vi "Servo.vi"() -> ()   [LabVIEW 2017]
uses:
  <vilib>/Platform/TimedLoop/XDataNode/timing_clust.ctl
  <vilib>/Platform/TimedLoop/XDataNode/nitl_modes.ctl
  <vilib>/Platform/TimedLoop/XDataNode/wakeup.ctl
  <vilib>/rvi/FXPMathLib/basic elements/FxpIntAccumulator/subVIs/nifxpmath_IntAccumulator_SimConfig.ctl
  <vilib>/rvi/Emulation/niFpgaGetClockAttributes.vi
  <vilib>/rvi/Emulation/niFpgaSctlEmulationGetInTimedLoop.vi
  <vilib>/rvi/Emulation/niFpgaEmulationReportErrorSimple.vi
  <vilib>/rvi/eio/common/nirviEmuTemplateMethod_errors.vi
  <vilib>/rvi/Emulation/niFpgaCriticalErrorInLSC.vi
  <vilib>/rvi/Analysis/common/codeGenErrors/XNode/niFpgaXNodeCodeGenErrorHandle.vi
  <vilib>/rvi/FXPMathLib/basic elements/FxpIntAccumulator/simVIs/DllFxpIntAccumulator_sub.vi
  <vilib>/eio/EIONode/EIONode.xnode
  <vilib>/rvi/Analysis/measure/dc-rms/XNode/niFpgaDC-RMS.xnode
  <vilib>/Platform/TimedLoop/XDataNode/XDataNode.xnode
  <vilib>/rvi/FXPMathLib/basic elements/FxpIntAccumulator/XNode/nifxpmath_IntAccumulator.xnode
  <vilib>/rvi/FXPMathLib/FxpMul/XNode/nifxpmath_Multiplier.xnode
  <vilib>/Platform/TimedLoop/XDataNode/XDNodeRunTimeDep.lvlib
  <vilib>/rvi/FXPMathLib/sim/FxpSim.dll
panel:
  out "Forward-Reverse":bool
  out "Continuous Mode Halt":bool
  out "Continuous Mode":bool
  out "raw period":i64
  out "period":i64
  in  "Sampling Interval for  1MHz\nFrequency (us)":u32=1
  in  "Offset":i64
  in  "Tacho Count(uSec) 2":u32 caption="Count(uSec)"
  in  "Tacho Count(uSec)":u32 caption="Count(uSec)"
  in  "Restart":bool
  in  "stop":bool
  in  "Halt":bool
  in  "Reset 2":bool
  out "Setpoint position":i64
  in  "Reset":bool
  out "Position shaft":i64
  in  "Forward/Reverse":bool
  in  "pulse width (ms)":u64=1500
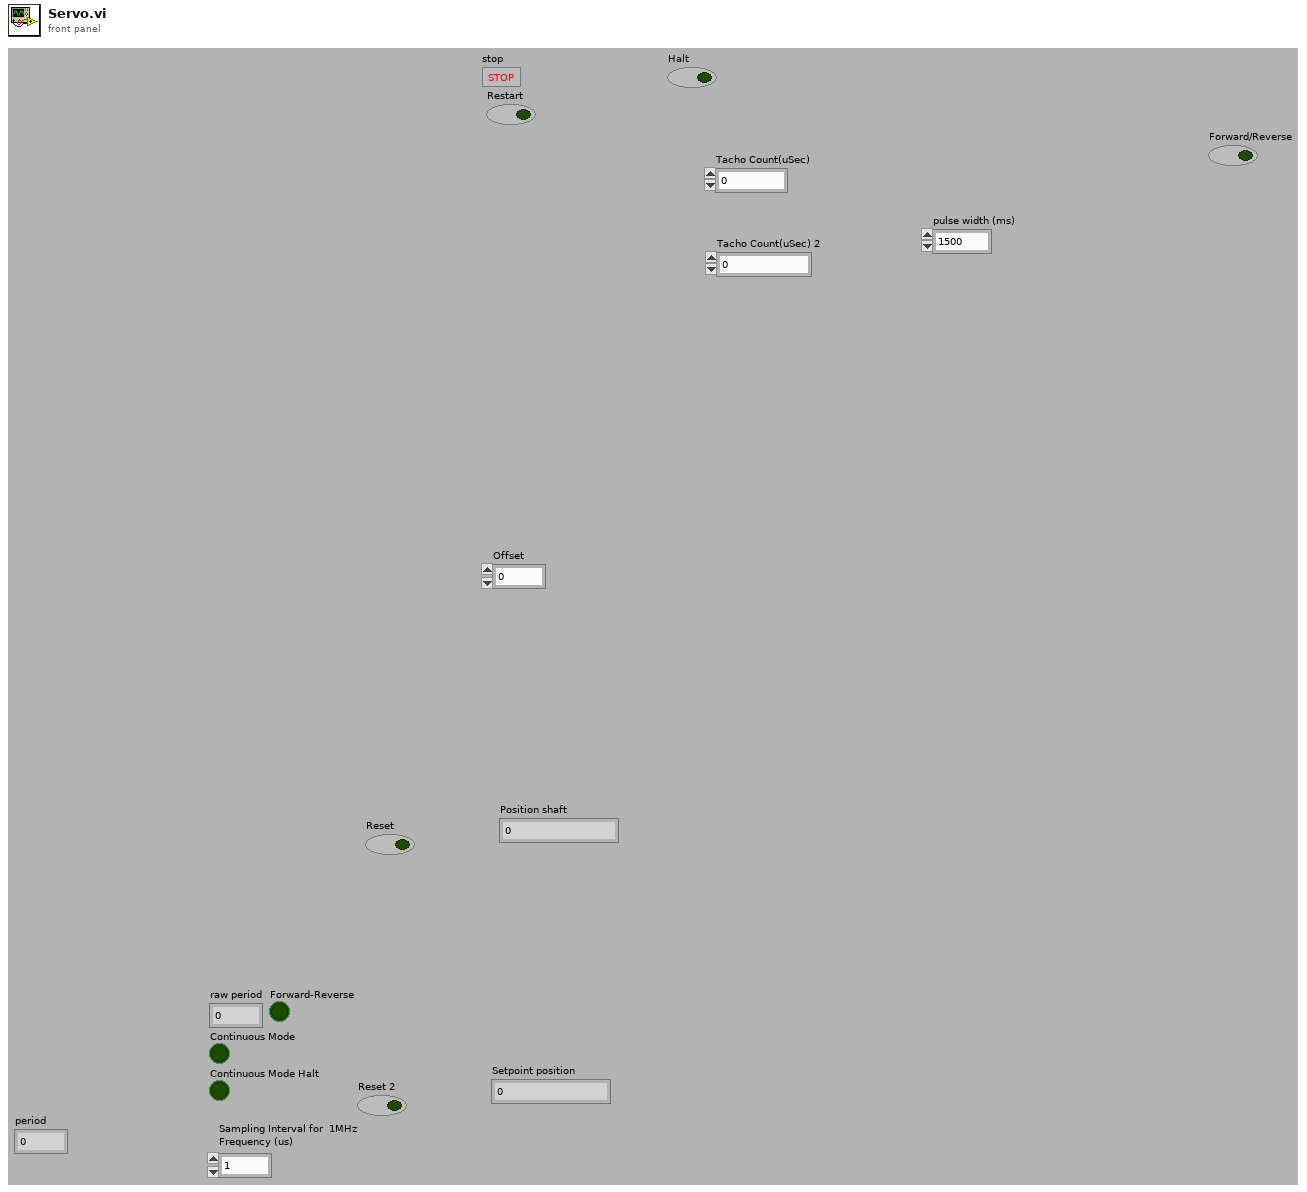
[diagram p1: front panel]
types:
  T1 = typedef "XDNodeRunTimeDep.lvlib/timing_clust.ctl" = cluster{"Expected End [f-1]":u64, "Actual End [f-1]":u64, "Finished Late? [f-1]":bool, "Expected End [i-1]":u64, "Actual End [i-1]":u64, "Finished Late? [i-1]":bool, "Expected Start [i]":u64, "Actual Start [i]":u64, "Expected Start [f]":u64, "Actual Start [f]":u64, "Source Name":string, "Structure Name":string, "Period":i64, "Deadline":i64, "Offset":i64, "Start":i64, "Priority":i32, "Timeout":i32, "Mode":T2, "Wakeup Reason":T3, "Error":errorcluster, "Source Type":string, "Secondary Source Type":string, "Global End Time":u64, "Global Start Time":u64, "Frame Duration":u64, "Iteration Duration":u64, "Assigned CPU":i32, "I/O Scan Engine Mode":u32}
  T2 = typedef "XDNodeRunTimeDep.lvlib/nitl_modes.ctl" = enum32{"No Change", "Process missed periods, maintain original phase", "Discard missed periods, maintain original phase", "Process missed periods, ignore original phase", "Discard missed periods, ignore original phase"}
  T3 = typedef "XDNodeRunTimeDep.lvlib/wakeup.ctl" = enum32{"Normal", "Aborted", "Asynchronous wakeup", "Timing source error", "Timed loop error", "Timeout"}
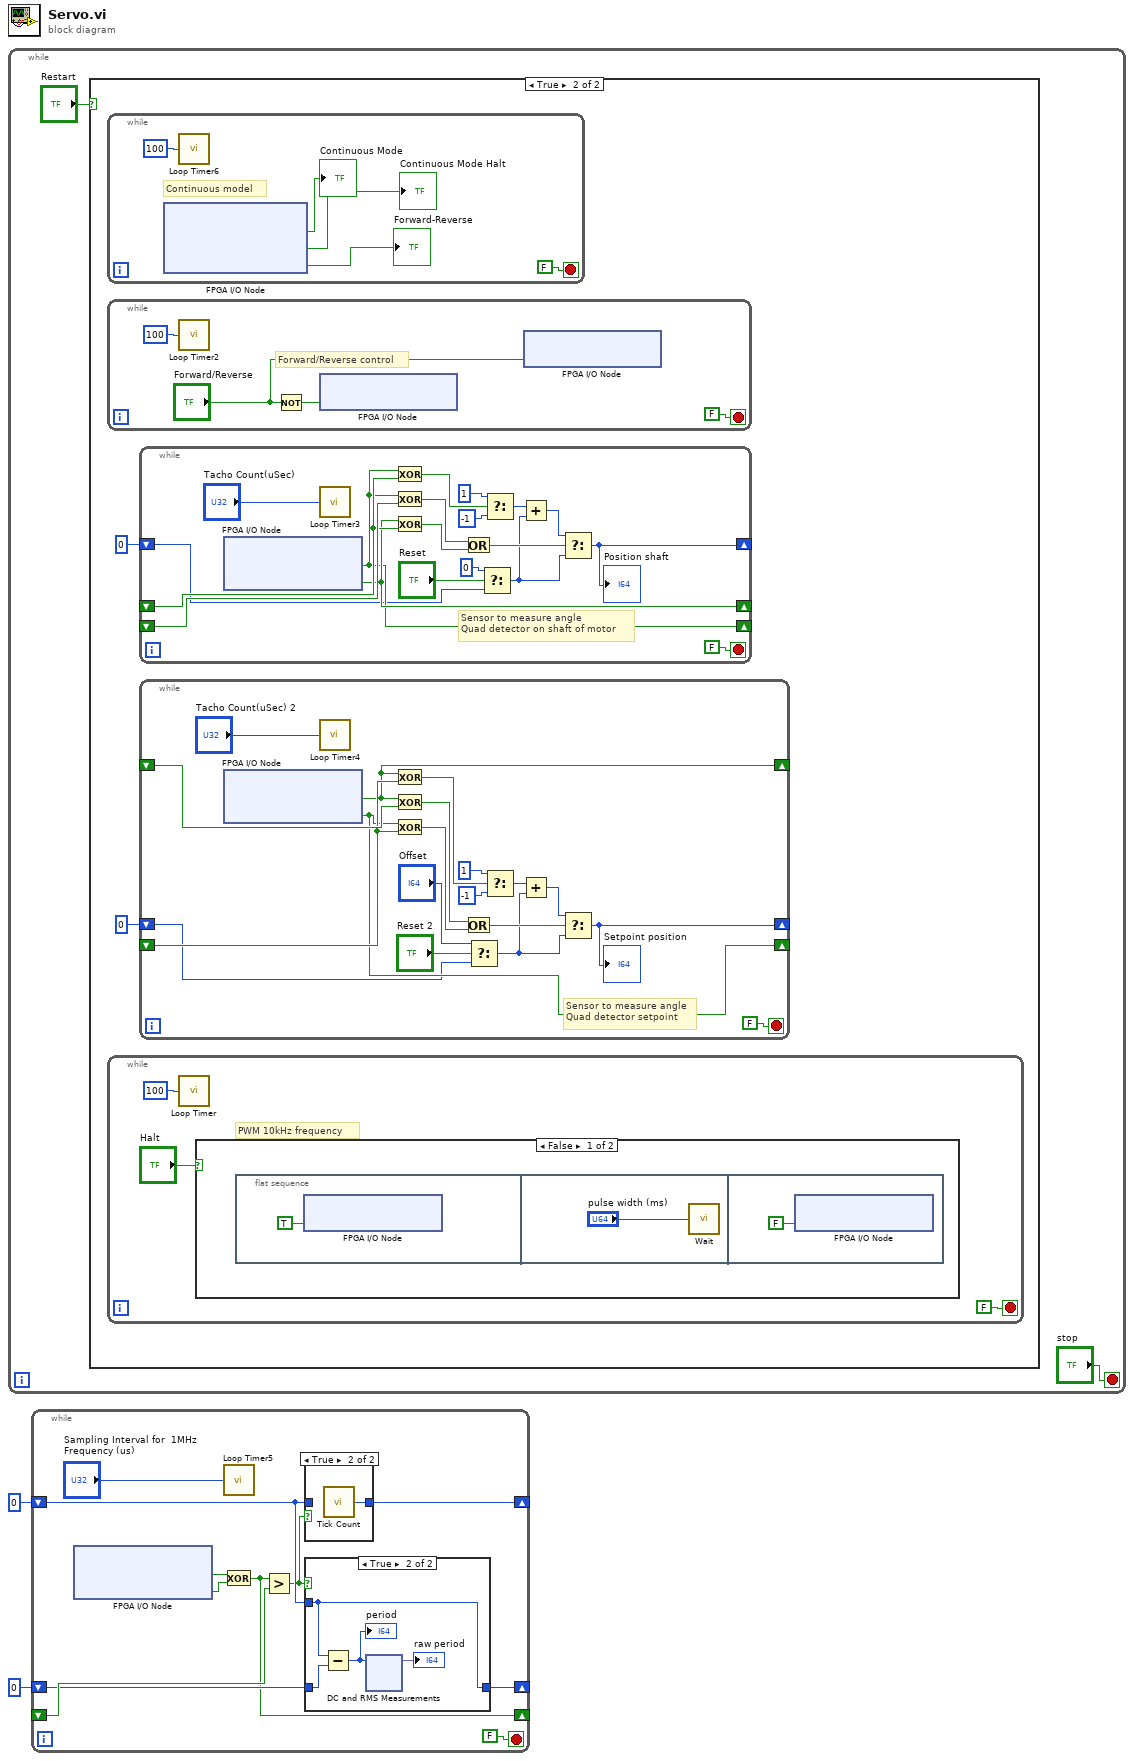
[diagram p0: block diagram]
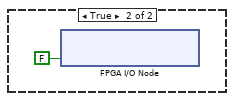
[diagram p5: hidden frame]
diagram:
  n1 = while {
    stop <- "stop" stop-if-true
    n2 = case shown="True" "Restart" {
      frame False {
      }
      frame True {
        n3 = while {
          stop <- FALSE stop-if-true
          # "Continuous model"
          n4 = xnode "FPGA I/O Node"() -> ("ConnectorB/DIO10"=→"Continuous Mode":bool, "ConnectorB/DIO9"=→"Continuous Mode Halt":bool, "ConnectorB/DIO8"=→"Forward-Reverse":bool)  [unwired: 3 in, 3 out]
          n5 = call "Loop Timer6"("Count(uSec)"=u32 100) -> ()  [unwired: 1 out]
        }
        n6 = while {
          stop <- FALSE stop-if-true
          # "Forward/Reverse control"
          n7 = call "Loop Timer2"("Count(uSec)"=u32 100) -> ()  [unwired: 1 out]
          n8 = Not(x="Forward/Reverse") -> (.not. x?=w52:bool)
          n9 = xnode "FPGA I/O Node"("ConnectorB/DIO1"=w52) -> ()  [unwired: 1 in, 1 out]
          n10 = xnode "FPGA I/O Node"("ConnectorB/DIO0"="Forward/Reverse") -> ()  [unwired: 1 in, 1 out]
        }
        n11 = while {
          stop <- FALSE stop-if-true
          # "PWM 10kHz frequency"
          n12 = call "Loop Timer"("Count(uSec)"=u32 100) -> ()  [unwired: 1 out]
          n13 = case shown="False" "Halt" {
            frame False {
              n14 = flat-sequence {
                frame #0 {
                  n15 = xnode "FPGA I/O Node"("ConnectorA/DIO7"=TRUE) -> ()  [unwired: 1 in, 1 out]
                }
                frame #1 {
                  n16 = call "Wait"("Count(uSec)"="pulse width (ms)") -> ()  [unwired: 1 out]
                }
                frame #2 {
                  n17 = xnode "FPGA I/O Node"("ConnectorA/DIO7"=FALSE) -> ()  [unwired: 1 in, 1 out]
                }
              }
            }
            frame True {
              n18 = xnode "FPGA I/O Node"("ConnectorA/DIO7"=FALSE) -> ()  [unwired: 1 in, 1 out]
            }
          }
        }
        n19 = while {
          shift-right: [w32] -> _
          shift-left: i64 0 ("Tick Count(Ticks)") -> [w33]
          shift-right: [w45] -> _
          shift-left: _ -> [w48]
          shift-right: [w46] -> _
          shift-left: _ -> [w47]
          stop <- FALSE stop-if-true
          # "Sensor to measure angle\nQuad detector on shaft of motor"
          n20 = xnode "FPGA I/O Node"() -> ("ConnectorA/DIO1"=w45:bool, "ConnectorA/DIO2"=w46:bool)  [unwired: 2 in, 2 out]
          n21 = call "Loop Timer3"("Count(uSec)"="Tacho Count(uSec)") -> ()  [unwired: 1 out]
          n22 = Exclusive Or(1:w47, 2:w45) -> (0:w42:bool)
          n23 = Exclusive Or(1:w48, 2:w45) -> (0:w44:bool)
          n24 = Exclusive Or(1:w47, 2:w46) -> (0:w43:bool)
          n25 = Or(x=w44, y=w43) -> (x .or. y?=w35:bool)
          n26 = Select(t=i16 0 ("Tick Count(Ticks)"), s="Reset", f=w33) -> (s? t:f=w34:i64)
          n27 = Select(t=i16 1 ("Tick Count(Ticks)"), s=w42, f=i16 -1 ("Tick Count(Ticks)")) -> (s? t:f=w37:i16)
          n28 = Add(x=w37, y=w34) -> (x+y=w36:i64)
          n29 = Select(t=w36, s=w35, f=w34) -> (s? t:f=w32:i64)
          "Position shaft" <- w32
        }
        n30 = while {
          shift-right: [w16] -> _
          shift-left: i64 0 ("Tick Count(Ticks)") -> [w15]
          shift-right: [w26] -> _
          shift-left: _ -> [w29]
          shift-right: [w27] -> _
          shift-left: _ -> [w28]
          stop <- FALSE stop-if-true
          # "Sensor to measure angle\nQuad detector setpoint"
          n31 = xnode "FPGA I/O Node"() -> ("ConnectorA/DIO3"=w26:bool, "ConnectorA/DIO4"=w27:bool)  [unwired: 2 in, 2 out]
          n32 = call "Loop Timer4"("Count(uSec)"="Tacho Count(uSec) 2") -> ()  [unwired: 1 out]
          n33 = Exclusive Or(1:w28, 2:w26) -> (0:w23:bool)
          n34 = Exclusive Or(1:w29, 2:w26) -> (0:w25:bool)
          n35 = Exclusive Or(1:w28, 2:w27) -> (0:w24:bool)
          n36 = Or(x=w25, y=w24) -> (x .or. y?=w17:bool)
          n37 = Select(t="Offset", s="Reset 2", f=w15) -> (s? t:f=w13:i64)
          n38 = Select(t=i16 1 ("Tick Count(Ticks)"), s=w23, f=i16 -1 ("Tick Count(Ticks)")) -> (s? t:f=w19:i16)
          n39 = Add(x=w19, y=w13) -> (x+y=w18:i64)
          n40 = Select(t=w18, s=w17, f=w13) -> (s? t:f=w16:i64)
          "Setpoint position" <- w16
        }
      }
    }
  }
  n41 = while {
    shift-right: [w61] -> _
    shift-left: _ -> [w71]
    shift-right: [w70] -> _
    shift-left: u32 0 ("Tick Count(Ticks)") -> [w66]
    shift-right: [w68] -> _
    shift-left: u32 0 ("Tick Count(Ticks)") -> [w69]
    stop <- FALSE stop-if-true
    n42 = xnode "FPGA I/O Node"() -> ("ConnectorA/DIO1"=w63:bool, "ConnectorA/DIO2"=w62:bool)  [unwired: 2 in, 2 out]
    n43 = call "Loop Timer5"("Count(uSec)"="Sampling Interval for  1MHz\nFrequency (us)") -> ()  [unwired: 1 out]
    n44 = Exclusive Or(1:w62, 2:w63) -> (0:w61:bool)
    n45 = Greater?(x=w61, y=w71) -> (0:w64:bool)
    n46 = case shown="True" w64 {
      tunnel: [w157 w158] -> w70
      tunnel: w66 -> [w157 _]
      frame False {
      }
      frame True {
        n47 = call "Tick Count"() -> ("Tick Count(uSec)"=w158:u32)
      }
    }
    n48 = case shown="True" w64 {
      tunnel: w69 -> [w72 w76]
      tunnel: [w72 w75] -> w68
      tunnel: w66 -> [_ w75]
      frame False {
      }
      frame True {
        n49 = Subtract(x=w75, y=w76) -> (x-y=w74:u32)
        "period" <- w74
        n50 = xnode "DC and RMS Measurements"("input data"=w74) -> ("DC"=→"raw period":fxp<+/-,32,33>)  [unwired: 1 in, 1 out]
      }
    }
  }
